vi "Core Action.vi"(8 "error in (no error)":errorcluster, 10 "SECS-II Class":refnum<class "SECS-II Class.lvclass">, 11 "18-Host Requests Equipment Process Program Directory in":refnum<class "18-Host Requests Equipment Process Program Directory.lvclass">) -> (0 "error out":errorcluster, 2 "SECS-II Class Out":refnum<class "SECS-II Class.lvclass">, 3 "18-Host Requests Equipment Process Program Directory out":refnum<class "18-Host Requests Equipment Process Program Directory.lvclass">)   [LabVIEW 2020, in "SECS Scenarios.lvlib" / "18-Host Requests Equipment Process Program Directory.lvclass"]
uses:
  18-Host Requests Equipment Process Program Directory.lvclass
  D:/Dropbox/SECS/SECS_GEM v1.1.0/Com/SECS Scenarios/Scenarios Class/Scenarios Class.lvclass
  SECS Communication/SECS-II Class/SECS-II Class.lvclass
  SECS Communication/S7 Message Class/S7 Message Class.lvclass
  D:/Dropbox/SECS/SECS_GEM v1.1.0/Com/SECS Communication/SECS-II Class/SECS-II Class.lvclass
  Scenarios Class/Reply State.ctl
  Scenarios Class/Scenarios Class.lvclass/Scenarios Class.ctl
  Scenarios Class/Write Reply State.vi
  Scenarios Class/Read HSMS Class.vi
  SECS Communication/HSMS Class/HSMS Class.lvclass
  Scenarios Class/Scenarios Class.lvclass
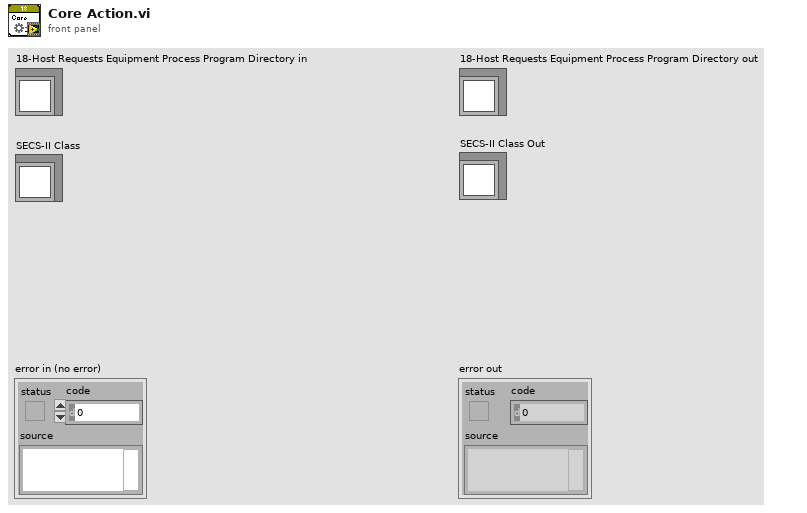
[diagram p1: front panel]
types:
  T1 = typedef "SECS Scenarios.lvlib/Scenarios Class.lvclass/Reply State.ctl" = enum16{"OK", "Illegal Data", "Unknown Stream", "Unknown Function", "Off-Line", "T3 Timeout", "Inner-Timeout"}
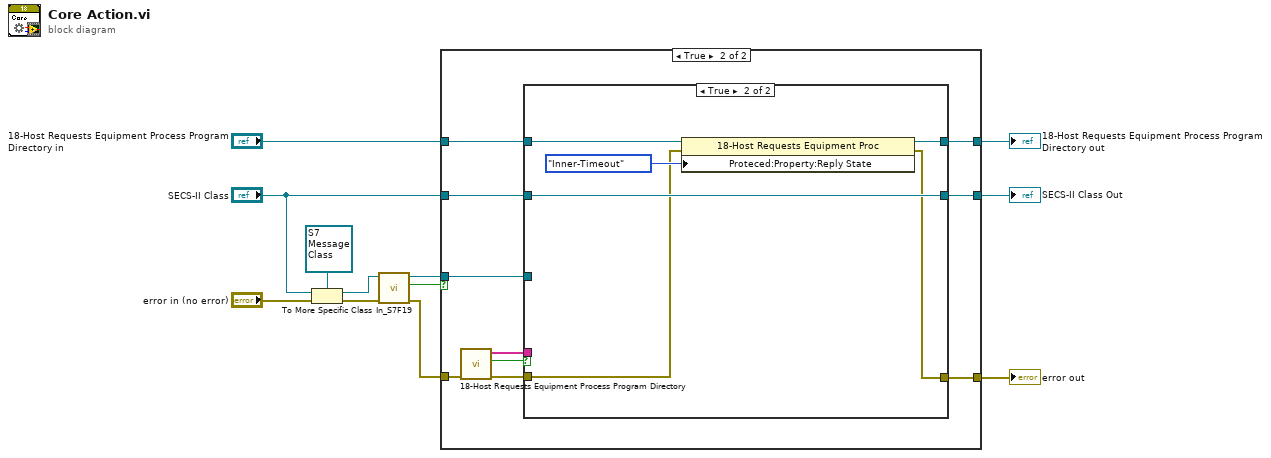
[diagram p0: block diagram]
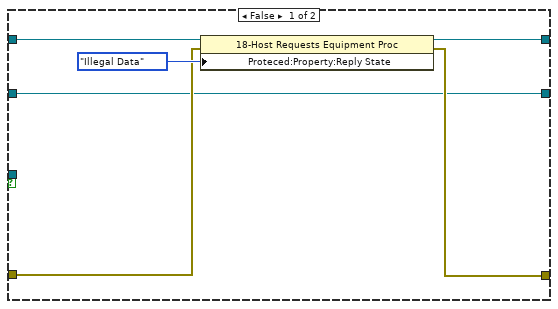
[diagram p2: hidden frame]
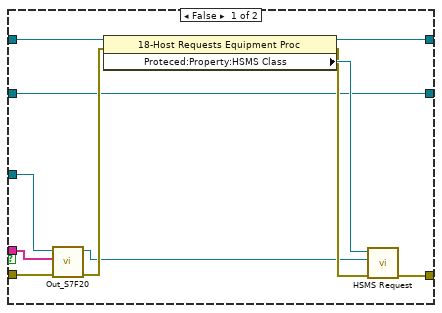
[diagram p3: hidden frame]
diagram:
  n1 = To More Specific Class(target class=refnum<class "S7 Message Class.lvclass"> refnum ("S7 Message Class in"), reference="SECS-II Class", error in="error in (no error)") -> (specific class reference=w10:refnum<class "S7 Message Class.lvclass">, error out=w11:errorcluster)
  n2 = call "In_S7F19.vi"("error in (no error)"=w11, "S7 Message Class in"=w10) -> ("error out"=w9:errorcluster, "OK?"=w3:bool, "S7 Message Class out"=w8:refnum<class "S7 Message Class.lvclass">)  [unwired: 7 in]
  n3 = case shown="True" w3 {
    tunnel: w9 -> [w15 w28]
    tunnel: w8 -> [_ w24]
    tunnel: "18-Host Requests Equipment Process Program Directory in" -> [w18 w23]
    tunnel: [w14 w22] -> w5
    tunnel: [w17 w21] -> w4
    tunnel: "SECS-II Class" -> [w13 w20]
    tunnel: [w13 w19] -> w1
    frame False {
      n4 = property class="18-Host Requests Equipment Proc"(reference=w18, error in=w15, "Proteced:Property:Reply State"=Reply_State."Illegal Data" ("Reply State")) -> (reference out=w17:refnum<class "18-Host Requests Equipment Process Program Directory.lvclass">, error out=w14:errorcluster)
    }
    frame True {
      n5 = call "18-Host Requests Equipment Process Program Directory.vi"("error in (no error)"=w28) -> ("error out"=w27:errorcluster, "Timeout?"=w26:bool, "PPID"=w25:string[])  [unwired: 8 in]
      n6 = case shown="True" w26 {
        tunnel: w23 -> [w39 w43]
        tunnel: w24 -> [w33 _]
        tunnel: [w36 w40] -> w22
        tunnel: [w35 w41] -> w21
        tunnel: w27 -> [w34 w42]
        tunnel: w25 -> [w30 _]
        tunnel: w20 -> [w29 w45]
        tunnel: [w29 w45] -> w19
        frame False {
          n7 = call "Out_S7F20.vi"("error in (no error)"=w34, "PPID"=w30, "S7 Message Class in"=w33) -> ("error out"=w32:errorcluster, "S7 Message Class out"=w31:refnum<class "S7 Message Class.lvclass">)  [unwired: 7 in]
          n8 = property class="18-Host Requests Equipment Proc"(reference=w39, error in=w32) -> (reference out=w35:refnum<class "18-Host Requests Equipment Process Program Directory.lvclass">, error out=w37:errorcluster, "Proteced:Property:HSMS Class"=w38:refnum<class "HSMS Class.lvclass">)
          n9 = call "HSMS Request.vi"("error in (no error)"=w37, "SECS-II Class In"=w31, "HSMS Class in"=w38) -> ("error out"=w36:errorcluster)  [unwired: 7 in, 1 out]
        }
        frame True {
          n10 = property class="18-Host Requests Equipment Proc"(reference=w43, error in=w42, "Proteced:Property:Reply State"=Reply_State."Inner-Timeout" ("Reply State")) -> (reference out=w41:refnum<class "18-Host Requests Equipment Process Program Directory.lvclass">, error out=w40:errorcluster)
        }
      }
    }
  }
  "error out" <- w5
  "18-Host Requests Equipment Process Program Directory out" <- w4
  "SECS-II Class Out" <- w1
